vi "solar_voy Register (Required).vi"(6 "Suppress Errors? (T)":bool=TRUE, 7 "Endian (BIG)":enum8{"BIG", "LITTLE"}(ring), 8 "error in (no error)":errorcluster, 9 "Override If Exists? (F)":bool, 10 "Target Name":string, 11 "Voyager Refnum in":T1) -> (0 "error out":errorcluster, 3 "Voyager Refnum out":T1)   [LabVIEW 2018]
uses:
  solar_voy_ctl Voyager Refnum.ctl
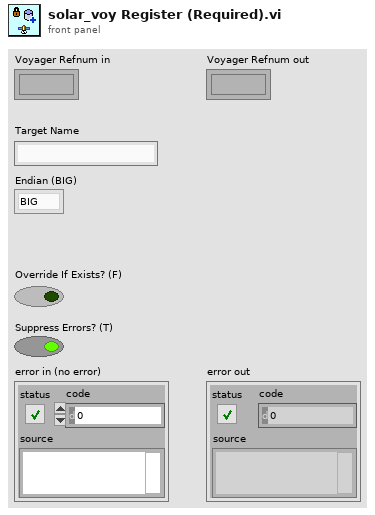
[diagram p1: front panel]
types:
  T1 = typedef "solar_voy_ctl Voyager Refnum.ctl" = refnum<k1>
  T2 = typedef "solar_voy_def_ctl PACKET.ctl" = cluster{"PACKET_ID":T3, "ENDIAN":enum8{"BIG", "LITTLE"}, "DESC":string, "HZRD":bool, "ITEMS":T4[], "NoExport":bool, "last_time":timestamp, "last_count":u32, "last_data":string}
  T3 = typedef "solar_voy_def_ctl PACKET_ID.ctl" = cluster{"ID":u16, "CMD":enum8{"CMD", "TLM"}, "TARGET":string, "PACKET":string}
  T4 = typedef "solar_voy_def_ctl ITEM.ctl" = cluster{"NAME":string, "OFFSET":i32, "SIZE":i32, "TYPE":T5, "EACH_SIZE":i32, "LVTYPE":T6, "MIN":dbl, "MAX":dbl, "DEFAULT":string, "DESC":string, "ID":bool, "MODIFIERS":variant, "last_value":variant}
  T5 = typedef "solar_voy_def_ctl ITEM TYPE.ctl" = enum8{"BLOCK", "INT", "UINT", "FLOAT", "STRING"}
  T6 = typedef "solar_type Item Type.ctl" = enum16{"NULL", "UNKNOWN", "CLUSTER", "I8", "I16", "I32", "I64", "U8", "U16", "U32", "U64", "U8_ENUM", "U16_ENUM", "U32_ENUM", "SGL", "DBL", "BOOLEAN", "STRING", "PATH", "VISA", "TAG", "TIME", "I8_1D", "I16_1D", "I32_1D", "I64_1D", "U8_1D", "U16_1D", "U32_1D", "U64_1D", "U8_ENUM_1D", "U16_ENUM_1D", "U32_ENUM_1D", "SGL_1D", "DBL_1D", "BOOLEAN_1D", "STRING_1D", "PATH_1D", "VISA_1D", "TAG_1D", "TIME_1D", "I8_2D", "I16_2D", "I32_2D", "I64_2D", "U8_2D", "U16_2D", "U32_2D", "U64_2D", "U8_ENUM_2D", "U16_ENUM_2D", "U32_ENUM_2D", "SGL_2D", "DBL_2D", "BOOLEAN_2D", "STRING_2D", "PATH_2D", "VISA_2D", "TAG_2D", "TIME_2D"}
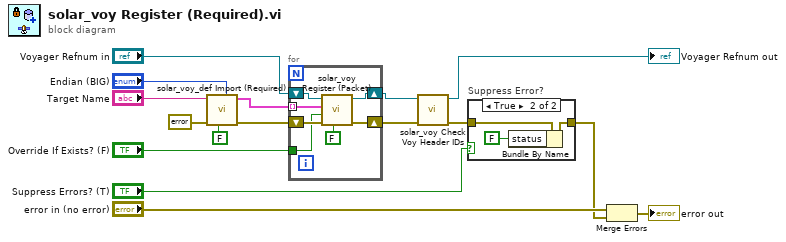
[diagram p0: block diagram]
diagram:
  n1 = call "solar_voy_def Import (Required).vi"("Endian (BIG)"="Endian (BIG)", "Suppress Errors? (T)"=FALSE, "error in (no error)"=errorcluster {"status"=FALSE, "code"=0, "source"=""} ("error out"), "Target Name"="Target Name") -> ("error out"=w11:errorcluster, "PACKETS (No HDR)"=w9:T2[])  [unwired: 6 in]
  n2 = for {
    shift-right: [w22] -> w4
    shift-left: w11 -> [w23]
    tunnel: w9 -> [w20] mode=indexing
    shift-right: [w18] -> w2
    shift-left: "Voyager Refnum in" -> [w19]
    tunnel: "Override If Exists? (F)" -> [w17]
    n3 = call "solar_voy Register (Packet).vi"("Suppress Errors? (T)"=FALSE, "error in (no error)"=w23, "Override If Exists? (F)"=w17, "PACKET (No HDR)"=w20, "Voyager Refnum in"=w19) -> ("error out"=w22:errorcluster, "Voyager Refnum out"=w18:T1)  [unwired: 5 in]
  }
  n4 = call "solar_voy Check Voy Header IDs.vi"("error in"=w4, "Voyager Refnum"=w2) -> ("Error out"=w3:errorcluster, "Voyager Refnum out"=→"Voyager Refnum out":T1)  [unwired: 8 in]
  n5 = case "Suppress Error?" shown="True" "Suppress Errors? (T)" {
    tunnel: w3 -> [w24 w27]
    tunnel: [w24 w26] -> w14
    frame False {
    }
    frame True {
      n6 = Bundle By Name(cluster=w27, "status"=FALSE) -> (w26:errorcluster)
    }
  }
  n7 = Merge Errors("error in (no error)", w14) -> (→"error out":errorcluster)
